vi "Write mayExplode_.vi"(8 "error in (no error)":errorcluster, 10 "mayExplode?":bool, 11 "Product in":refnum<class "Product.lvclass">) -> (0 "error out":errorcluster, 3 "Product out":refnum<class "Product.lvclass">)   [LabVIEW 2018, in "Product.lvclass"]
uses:
  Product.lvclass
  Product.lvclass/Product.ctl
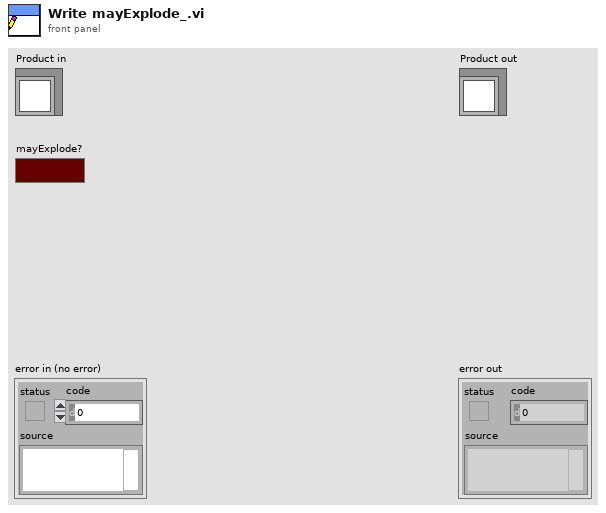
[diagram p1: front panel]
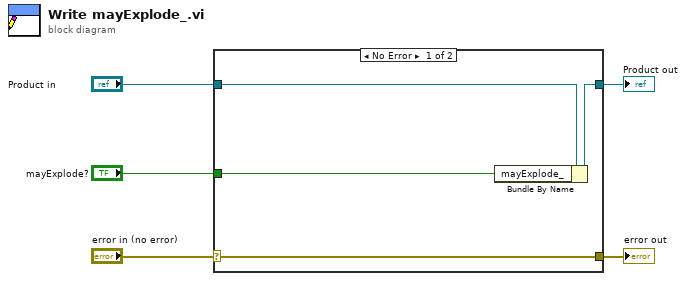
[diagram p0: block diagram]
diagram:
  n1 = case shown="No Error" "error in (no error)" {
    selector: "error in (no error)" -> [w9 w10]
    tunnel: [w9 w10] -> w4
    tunnel: [w7 w11] -> w2
    tunnel: "Product in" -> [w8 w11]
    tunnel: "mayExplode?" -> [w6 _]
    frame No Error {
      n2 = Bundle By Name(cluster=w8, "mayExplode_"=w6) -> (w7:refnum<class "Product.lvclass">)
    }
    frame Error {
    }
  }
  "error out" <- w4
  "Product out" <- w2
